vi "Relay_tb.vi"() -> ()   [LabVIEW 2018]
panel:
  in  "IN1":bool
  in  "IN2":bool
  in  "stop (F)":bool
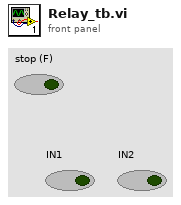
[diagram p1: front panel]
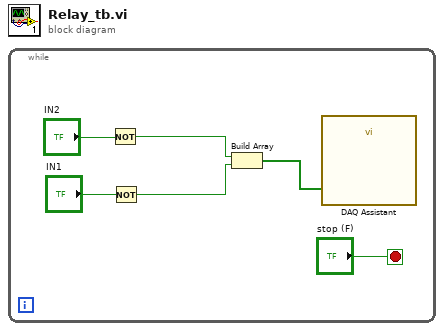
[diagram p0: block diagram]
diagram:
  n1 = while {
    stop <- "stop (F)" stop-if-true
    n2 = Not(x="IN2") -> (.not. x?=w2:bool)
    n3 = Not(x="IN1") -> (.not. x?=w1:bool)
    n4 = Build Array(w2, w1) -> (w5:bool[])
    n5 = call "DAQ Assistant"("data"=w5) -> ()  [unwired: 17 in, 2 out]
  }
